vi "CloseScope.vi"(1 "IVI Logical Name":refnum<k15>) -> (0 "error out":errorcluster {"code" format="%.0x"})   [LabVIEW 2012]
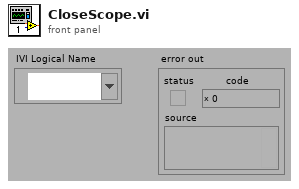
[diagram p1: front panel]
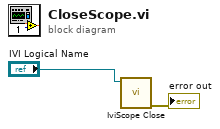
[diagram p0: block diagram]
diagram:
  n1 = call <vilib>:"IviScope Close.vi"("instrument handle"="IVI Logical Name") -> ("error out"=→"error out":errorcluster)  [unwired: 1 in, 9 out]
